vi "Test Matches.vi"() -> ()   [LabVIEW 2020]
uses:
  <vilib>/regexp/Match Regular Expression.xnode
panel:
  out "result string":string
  out "Description":string
  out "Status":string
  out "after match":string
  in  "String":string="{\"code\":\"not found\",\"message\":\"failed to initialize execute state: could not find bucket \\\"Test1\\\"\"}"
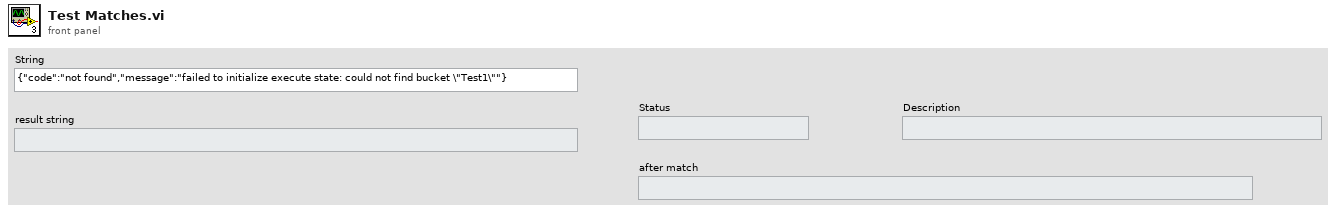
[diagram p1: front panel]
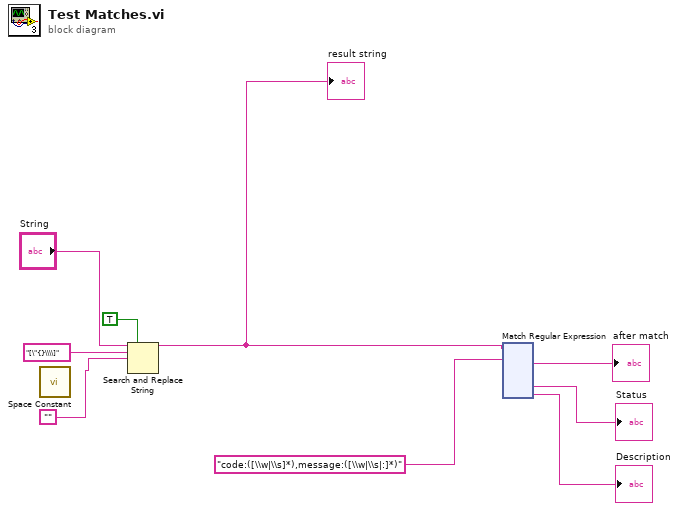
[diagram p0: block diagram]
diagram:
  n1 = call <vilib>:"Space Constant.vi"() -> ()  [unwired: 1 out]
  n2 = Search and Replace String(replace all?=TRUE ("replace all? (F)"), input string="String", search string="[\"{}\\\\]", replace string="") -> (result string=w1:string)  [unwired: 4 in, 3 out]
  "result string" <- w1
  n3 = xnode "Match Regular Expression"("input string"=w1, "regular expression"="code:([\\w|\\s]*),message:([\\w|\\s|:]*)") -> ("after match"=→"after match":string, "submatch 1"=→"Status":string, "submatch 2"=→"Description":string)  [unwired: 4 in, 4 out]
